vi "断电保存全局.vi"() -> ()   [LabVIEW 2016]
panel:
  in  "超标留样型号":T1(ring)
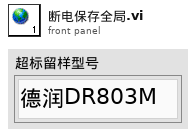
[diagram p1: front panel]
types:
  T1 = enum16{"德润DR803M", "德润DR803L", "德润DR803F", "科盛超标留样"}
diagram:
